vi "setConfiguration.vi"(8 "error in (no error)":errorcluster, 10 "configuration":T2={"exposure_time_s"=nan, "delay_time_s"=nan, "roi"={"x0"=18446744073709551615, "y0"=18446744073709551615, "x1"=18446744073709551615, "y1"=18446744073709551615}, "timestamp_mode"=65535, "pixelrate"=4294967295, "conversion_factor"=0.7, "trigger_mode"=65535, "acquire_mode"=65535, "acquire_sequence_number"=1, "metadata_mode"=65535, "noisefilter_mode"=65535, "pixel_format"=0, "binning"={"vert"=0, "horz"=0, "mode"=0}, "auto_exposure"={"region"=0, "min_exposure_s"=0.001, "max_exposure_s"=0.1}} {"conversion_factor" format="%.2g"; "auto_exposure"."region" items=["balanced", "center_based", "corner_based", "full", "custom"]; "binning"."mode" items=["sum", "average"]; "noisefilter_mode" items=["Undefined"=65535, "OFF"=0, "ON"=1]; "exposure_time_s" format="%#_6f"; "timestamp_mode" items=["Undefined"=65535, "OFF"=0, "Binary"=1, "Binary+ASCII"=2, "ASCII"=3]; "acquire_mode" items=["Undefined"=65535, "auto"=0, "external"=1, "external modulate"=2]; "trigger_mode" items=["Undefined"=65535, "auto sequence"=0, "software trigger"=1, "external exposure start & software trigger"=2, "external exposure control"=3, "external synchronized"=4, "fast external exposure control"=5, "external CDS control"=6, "slow external exposure control"=7, "external synchronized HDSDI"=258]; "metadata_mode" items=["Undefined"=65535, "OFF"=0, "ON"=1]}, 11 "Camera in":refnum<class "Camera.lvclass">) -> (0 "error out":errorcluster, 3 "Camera out":refnum<class "Camera.lvclass">)   [LabVIEW 2019, in "Camera.lvclass"]
doc: "Sets a new coniguration to the camera."
uses:
  Camera.lvclass
  Camera.lvclass/Camera.ctl
  pco.sdk/TimingControl/TimingControl.lvlib
  pco.sdk/ImageSensor/ImageSensor.lvlib
  pco.sdk/RecordingControl/RecordingControl.lvlib
  pco.sdk/CameraDescription/CameraDescription.lvlib
  pco.sdk/GeneralCameraControl/GeneralCameraControl.lvlib
  Controls/binning.ctl
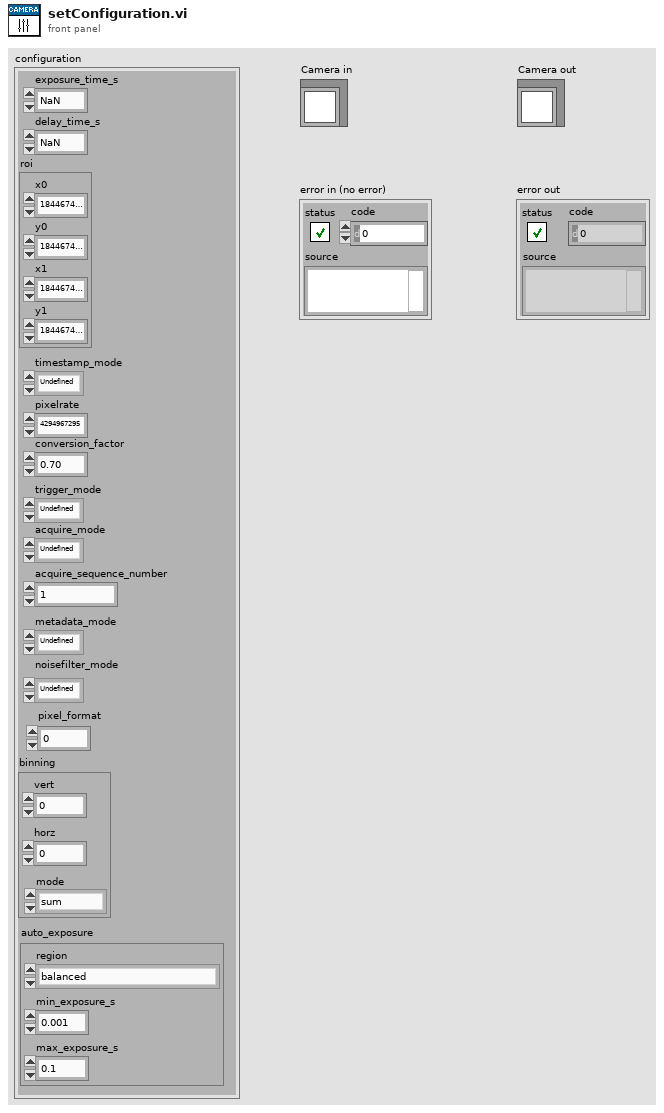
[diagram p1: front panel]
types:
  T1 = typedef "Camera.lvclass/binning.ctl" = cluster{"vert":u16, "horz":u16, "mode":u16}
  T2 = cluster{"exposure_time_s":dbl, "delay_time_s":dbl, "roi":cluster{"x0":u64, "y0":u64, "x1":u64, "y1":u64}, "timestamp_mode":u16, "pixelrate":u32, "conversion_factor":sgl, "trigger_mode":u16, "acquire_mode":u16, "acquire_sequence_number":u32, "metadata_mode":u16, "noisefilter_mode":u16, "pixel_format":u32, "binning":T1, "auto_exposure":cluster{"region":u16, "min_exposure_s":dbl, "max_exposure_s":dbl}}
  T3 = cluster{"region":u16, "min_exposure_s":dbl, "max_exposure_s":dbl}
  T4 = cluster{"wSensorTypeDESC":u16, "wSensorSubTypeDESC":u16, "wMaxHorzResStdDESC":u16, "wMaxVertResStdDESC":u16, "wMaxHorzResExtDESC":u16, "wMaxVertResExtDESC":u16, "wDynResDESC":u16, "wMaxBinHorzDESC":u16, "wBinHorzSteppingDESC":u16, "wMaxBinVertDESC":u16, "wBinVertSteppingDESC":u16, "wRoiHorStepsDESC":u16, "wRoiVertStepsDESC":u16, "wNumADCsDESC":u16, "wMinSizeHorzDESC":u16, "dwPixelRateDESC":u32[], "wConvFactDESC":u16[], "sCoolingSetpoints":i16[], "wSoftRoiHorStepsDESC":u16, "wSoftRoiVertStepsDESC":u16, "wIRDESC":u16, "wMinSizeVertDESC":u16, "dwMinDelayDESC":u32, "dwMaxDelayDESC":u32, "dwMinDelayStepDESC":u32, "dwMinExposureDESC":u32, "dwMaxExposureDESC":u32, "dwMinExposureStepDESC":u32, "dwMinDelayIRDESC":u32, "dwMaxDelayIRDESC":u32, "dwMinExposureIRDESC":u32, "dwMaxExposureIRDESC":u32, "wTimeTableDESC":u16, "wDoubleImageDESC":u16, "sMinCoolSetDESC":i16, "sMaxCoolSetDESC":i16, "sDefaultCoolSetDESC":i16, "wPowerDownModeDESC":u16, "wOffsetRegulationDESC":u16, "wColorPatternDESC":u16, "wPatternTypeDESC":u16, "wNumCoolingSetpoints":u16, "dwGeneralCapsDESC1":u32, "dwGeneralCapsDESC2":u32, "dwExtSyncFrequency":u32[], "dwGeneralCapsDESC3":u32, "dwGeneralCapsDESC4":u32}
  T5 = enum16{"SETUP_TYPE_SHUTTERMODE", "SETUP_TYPE_PIXELFORMAT", "SETUP_TYPE_SENSOR_DYNRES"}
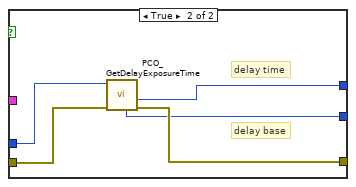
[diagram p4: hidden frame]
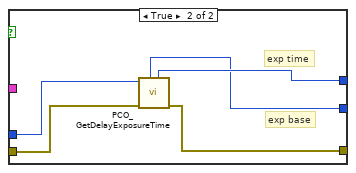
[diagram p5: hidden frame]
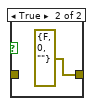
[diagram p9: hidden frame]
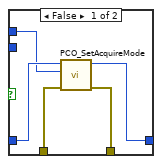
[diagram p12: hidden frame]
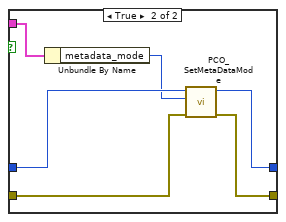
[diagram p13: hidden frame]
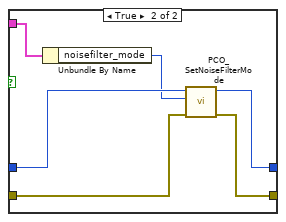
[diagram p14: hidden frame]
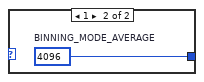
[diagram p16: hidden frame]
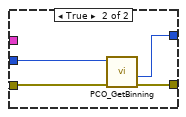
[diagram p17: hidden frame]
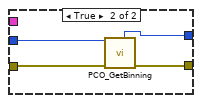
[diagram p18: hidden frame]
diagram:
  n1 = case shown="No Error" "error in (no error)" {
    selector: "error in (no error)" -> [w10 w448]
    tunnel: [w13 w448] -> w4
    tunnel: [w12 w447] -> w2
    tunnel: "Camera in" -> [w11 w447]
    tunnel: "configuration" -> [w6 _]
    frame No Error {
      n2 = call-dynamic "isRecording.vi"("Camera in"=w11, "error in (no error)"=w10) -> ("Camera out"=w7:refnum<class "Camera.lvclass">, "recording"=w9:bool, "error out"=w8:errorcluster)  [unwired: 11 in]
      n3 = case shown="False" w9 {
        tunnel: [w18 errorcluster {"status"=TRUE, "code"=-2146029534, "source"="Cannot set configuration\nif recording is running!"} ("error constant")] -> w13
        tunnel: [w17 w445] -> w12
        tunnel: w8 -> [w16 _]
        tunnel: w7 -> [w14 w445]
        tunnel: w6 -> [w15 _]
        frame False {
          n4 = Unbundle By Name(w14) -> ("camera_handle"=w19:u64)
          n5 = Not Equal To 0?(x=w19) -> (x != 0?=w20:bool)
          n6 = case shown="True" w20 {
            tunnel: [errorcluster {"status"=TRUE, "code"=1, "source"="In set_configuration:\nCamera handle is zero"} ("error constant") w36] -> w18
            tunnel: w19 -> [_ w63]
            tunnel: w16 -> [_ w62]
            tunnel: w14 -> [w21 w27]
            tunnel: [w21 w28] -> w17
            tunnel: w15 -> [_ w61]
            frame False {
            }
            frame True {
              n7 = flat-sequence {
                tunnel: w63 -> [w70]
                tunnel: w62 -> [w67]
                tunnel: w61 -> [w66]
                tunnel: [w66] -> w60
                tunnel: [w65] -> w59
                tunnel: [w64] -> w58
                tunnel: w60 -> [w117]
                tunnel: w59 -> [w116]
                tunnel: w58 -> [w115]
                tunnel: [w117] -> w57
                tunnel: [w114] -> w56
                tunnel: [w113] -> w55
                tunnel: w57 -> [w145]
                tunnel: w56 -> [w144]
                tunnel: w55 -> [w143]
                tunnel: w27 -> [w150]
                tunnel: [w145] -> w54
                tunnel: [w142] -> w53
                tunnel: [w141] -> w52
                tunnel: w54 -> [w165]
                tunnel: w53 -> [w164]
                tunnel: w52 -> [w163]
                tunnel: [w165] -> w51
                tunnel: [w162] -> w49
                tunnel: [w161] -> w47
                tunnel: w51 -> [w188]
                tunnel: [w188] -> w50
                tunnel: w49 -> [w187]
                tunnel: [w185] -> w48
                tunnel: w47 -> [w186]
                tunnel: [w184] -> w46
                tunnel: w50 -> [w205]
                tunnel: w48 -> [w208]
                tunnel: w46 -> [w207]
                tunnel: w27 -> [w206]
                tunnel: [w205] -> w45
                tunnel: [w204] -> w44
                tunnel: [w203] -> w43
                tunnel: w27 -> [w200]
                tunnel: w45 -> [w242]
                tunnel: w27 -> [w247]
                tunnel: w44 -> [w246]
                tunnel: w43 -> [w245]
                tunnel: [w242] -> w42
                tunnel: [w241] -> w41
                tunnel: [w240] -> w40
                tunnel: w42 -> [w271]
                tunnel: w41 -> [w273]
                tunnel: w40 -> [w272]
                tunnel: [w271] -> w39
                tunnel: [w270] -> w38
                tunnel: [w269] -> w37
                tunnel: w27 -> [w262]
                tunnel: w39 -> [w284]
                tunnel: w38 -> [w300]
                tunnel: w37 -> [w299]
                tunnel: [w284] -> w35
                tunnel: [w296] -> w34
                tunnel: [w295] -> w33
                tunnel: w27 -> [w293]
                tunnel: w35 -> [w345]
                tunnel: w34 -> [w347]
                tunnel: w33 -> [w342]
                tunnel: w27 -> [w346]
                tunnel: [w340] -> w23
                tunnel: [w345] -> w32
                tunnel: [w347] -> w31
                tunnel: [w341] -> w30
                tunnel: w32 -> [w353]
                tunnel: w31 -> [w361]
                tunnel: w30 -> [w360]
                tunnel: [w353] -> w26
                tunnel: [w352] -> w25
                tunnel: [w348] -> w24
                tunnel: [w431] -> w29
                tunnel: [w434] -> _
                tunnel: w26 -> [w434]
                tunnel: w25 -> [w432]
                tunnel: w24 -> [w433]
                tunnel: w23 -> [w430]
                frame #0 {
                  w73 = nan
                  # "Set Delay and Exposure Time"
                  n8 = Unbundle By Name(w66) -> ("exposure_time_s"=w74:dbl, "delay_time_s"=w72:dbl)
                  n9 = Not Equal?(x=w73, y=w74) -> (x != y?=w68:bool)
                  n10 = Not Equal?(x=w73, y=w72) -> (x != y?=w69:bool)
                  n11 = Or(x=w68, y=w69) -> (x .or. y?=w71:bool)
                  n12 = case shown="True" w71 {
                    tunnel: w66 -> [_ w88]
                    tunnel: w70 -> [w76 w86]
                    tunnel: w69 -> [_ w89]
                    tunnel: w68 -> [_ w91]
                    tunnel: w67 -> [w75 w87]
                    tunnel: [w76 w78] -> w65
                    tunnel: [w75 w77] -> w64
                    frame False {
                    }
                    frame True {
                      # "If delay time is nan"
                      # "If exp time is nan"
                      n13 = Not(x=w89) -> (.not. x?=w90:bool)
                      n14 = Not(x=w91) -> (.not. x?=w92:bool)
                      n15 = case shown="False" w90 {
                        tunnel: w86 -> [_ w101]
                        tunnel: w88 -> [w96 _]
                        tunnel: [w95 w99] -> w80
                        tunnel: [w94 w98] -> w79
                        tunnel: w87 -> [w93 w102]
                        tunnel: [w93 w100] -> w83
                        frame False {
                          # "delay base"
                          # "delay time"
                          n16 = Unbundle By Name(w96) -> ("delay_time_s"=w97:dbl)
                          n17 = call "calcTimeBase.vi"("time"=w97) -> ("base_calculated"=w94:u16, "time_calculated"=w95:u32)  [unwired: 9 in]
                        }
                        frame True {
                          # "delay base"
                          # "delay time"
                          n18 = call "PCO_GetDelayExposureTime.vi"("error in (no error)"=w102, "ph"=w101) -> ("error out"=w100:errorcluster, "dwDelay"=w99:u32, "wTimeBaseDelay"=w98:u16)  [unwired: 3 in, 4 out]
                        }
                      }
                      n19 = case shown="False" w92 {
                        tunnel: w86 -> [_ w112]
                        tunnel: w88 -> [w107 _]
                        tunnel: [w105 w109] -> w82
                        tunnel: [w104 w108] -> w81
                        tunnel: w87 -> [w103 w111]
                        tunnel: [w103 w110] -> w84
                        frame False {
                          # "exp base"
                          # "exp time"
                          n20 = Unbundle By Name(w107) -> ("exposure_time_s"=w106:dbl)
                          n21 = call "calcTimeBase.vi"("time"=w106) -> ("base_calculated"=w104:u16, "time_calculated"=w105:u32)  [unwired: 9 in]
                        }
                        frame True {
                          # "exp base"
                          # "exp time"
                          n22 = call "PCO_GetDelayExposureTime.vi"("error in (no error)"=w111, "ph"=w112) -> ("error out"=w110:errorcluster, "dwExposure"=w109:u32, "wTimeBaseExposure"=w108:u16)  [unwired: 3 in, 4 out]
                        }
                      }
                      n23 = Merge Errors(w84, w83) -> (w85:errorcluster)
                      n24 = call "PCO_SetDelayExposureTime.vi"("wTimeBaseExposure"=w81, "wTimeBaseDelay"=w79, "error in (no error)"=w85, "dwExposure"=w82, "dwDelay"=w80, "ph"=w86) -> ("error out"=w77:errorcluster, "ph out"=w78:u64)  [unwired: 3 in, 1 out]
                    }
                  }
                }
                frame #1 {
                  w127 = u64 18446744073709551615
                  # "Set ROI"
                  n25 = Unbundle By Name(w117) -> ("roi.x0"=w126:u64, "roi.y0"=w125:u64, "roi.x1"=w124:u64, "roi.y1"=w123:u64)
                  n26 = Not Equal?(x=w127, y=w126) -> (x != y?=w122:bool)
                  n27 = Not Equal?(x=w127, y=w125) -> (x != y?=w121:bool)
                  n28 = Not Equal?(x=w127, y=w124) -> (x != y?=w120:bool)
                  n29 = Not Equal?(x=w127, y=w123) -> (x != y?=w119:bool)
                  n30 = Compound Arithmetic op=AND(w122, w121, w120, w119) -> (w118:bool)
                  n31 = case shown="True" w118 {
                    tunnel: w117 -> [_ w136]
                    tunnel: w116 -> [w129 w134]
                    tunnel: w115 -> [w128 w135]
                    tunnel: [w129 w138] -> w114
                    tunnel: [w128 w137] -> w113
                    frame False {
                    }
                    frame True {
                      n32 = Unbundle By Name(w136) -> ("roi.x0"=w133:u64, "roi.y0"=w132:u64, "roi.x1"=w131:u64, "roi.y1"=w130:u64)
                      n33 = call "PCO_SetROI.vi"("ph"=w134, "wRoiX0"=w133, "wRoiX1"=w131, "error in (no error)"=w135, "wRoiY0"=w132, "wRoiY1"=w130) -> ("ph out"=w138:u64, "error out"=w137:errorcluster)  [unwired: 7 in, 1 out]
                    }
                  }
                }
                frame #2 {
                  w139 = u32 256 ("camera_description.dwGeneralCapsDESC1")
                  # "Set Timestamp Mode"
                  # "GENERALCAPS1_NO_TIMESTAMP"
                  n34 = Unbundle By Name(w150) -> ("dwGeneralCapsDESC1"=w149:u32)
                  n35 = Unbundle By Name(w145) -> ("timestamp_mode"=w151:u16)
                  n36 = Not Equal?(x=u16 65535 ("timestamp_mode"), y=w151) -> (x != y?=w148:bool)
                  n37 = And(x=w149, y=w139) -> (x .and. y?=w140:u32)
                  n38 = Not Equal?(x=w140, y=w139) -> (x != y?=w147:bool)
                  n39 = And(x=w148, y=w147) -> (x .and. y?=w146:bool)
                  n40 = case shown="True" w146 {
                    tunnel: w145 -> [_ w160]
                    tunnel: w144 -> [w154 w159]
                    tunnel: w143 -> [w153 w158]
                    tunnel: [w154 w156] -> w142
                    tunnel: [w153 w155] -> w141
                    frame False {
                    }
                    frame True {
                      n41 = Unbundle By Name(w160) -> ("timestamp_mode"=w157:u16)
                      n42 = call "PCO_SetTimestampMode.vi"("error in (no error)"=w158, "wTimeStampMode"=w157, "ph"=w159) -> ("error out"=w155:errorcluster, "ph out"=w156:u64)  [unwired: 6 in, 1 out]
                    }
                  }
                }
                frame #3 {
                  # "Set Pixelrate"
                  n43 = Unbundle By Name(w165) -> ("pixelrate"=w168:u32)
                  n44 = Not Equal?(x=u32 4294967295 ("pixelrate"), y=w168) -> (x != y?=w166:bool)
                  n45 = case shown="True" w166 {
                    tunnel: w165 -> [_ w181]
                    tunnel: w164 -> [w170 w180]
                    tunnel: w163 -> [w169 w178]
                    tunnel: [w170 w172] -> w162
                    tunnel: [w169 w171] -> w161
                    frame False {
                    }
                    frame True {
                      w175 = -2147479520 ("ErrorMessage")
                      # "Ignore\nPCO_ERROR_FIRMWARE_NOT_SUPPORTED"
                      n46 = Unbundle By Name(w181) -> ("pixelrate"=w179:u32)
                      n47 = call "PCO_SetPixelRate.vi"("error in (no error)"=w178, "dwPixelRate"=w179, "ph"=w180) -> ("error out"=w173:errorcluster, "ErrorMessage"=w177:i32, "ph out"=w172:u64)  [unwired: 6 in]
                      n48 = And(x=w177, y=w175) -> (x .and. y?=w176:i32)
                      n49 = Equal?(x=w176, y=w175) -> (x = y?=w174:bool)
                      n50 = case shown="False" w174 {
                        tunnel: w173 -> [w182 _]
                        tunnel: [w182 errorcluster {"status"=FALSE, "code"=0, "source"=""} ("error out")] -> w171
                        frame False {
                        }
                        frame True {
                        }
                      }
                    }
                  }
                }
                frame #4 {
                  # "Set Trigger Mode"
                  n51 = Unbundle By Name(w188) -> ("trigger_mode"=w190:u16)
                  n52 = Not Equal?(x=u16 65535 ("timestamp_mode"), y=w190) -> (x != y?=w189:bool)
                  n53 = case shown="True" w189 {
                    tunnel: w188 -> [_ w199]
                    tunnel: w187 -> [w193 w198]
                    tunnel: w186 -> [w192 w197]
                    tunnel: [w193 w195] -> w185
                    tunnel: [w192 w194] -> w184
                    frame False {
                    }
                    frame True {
                      n54 = Unbundle By Name(w199) -> ("trigger_mode"=w196:u16)
                      n55 = call "PCO_SetTriggerMode.vi"("error in (no error)"=w197, "wTriggerMode"=w196, "ph"=w198) -> ("error out"=w194:errorcluster, "ph out"=w195:u64)  [unwired: 6 in, 1 out]
                    }
                  }
                }
                frame #5 {
                  w201 = u32 512 ("camera_description.dwGeneralCapsDESC1")
                  # "Set Acquire Mode"
                  # "GENERALCAPS1_NO_ACQUIREMODE"
                  n56 = Unbundle By Name(w206) -> ("dwGeneralCapsDESC1"=w212:u32)
                  n57 = Unbundle By Name(w205) -> ("acquire_mode"=w213:u16)
                  n58 = Not Equal?(x=u16 65535 ("timestamp_mode"), y=w213) -> (x != y?=w211:bool)
                  n59 = And(x=w212, y=w201) -> (x .and. y?=w202:u32)
                  n60 = Not Equal?(x=w202, y=w201) -> (x != y?=w210:bool)
                  n61 = And(x=w211, y=w210) -> (x .and. y?=w209:bool)
                  n62 = case shown="True" w209 {
                    tunnel: w205 -> [_ w228]
                    tunnel: w208 -> [w216 w227]
                    tunnel: w207 -> [w215 w226]
                    tunnel: [w216 w224] -> w204
                    tunnel: [w215 w223] -> w203
                    tunnel: w200 -> [_ w222]
                    frame False {
                    }
                    frame True {
                      w219 = u32 2097152 ("y")
                      # "GENERALCAPS1_EXT_ACQUIRE"
                      n63 = Unbundle By Name(w222) -> ("dwGeneralCapsDESC1"=w221:u32)
                      n64 = Unbundle By Name(w228) -> ("acquire_mode"=w225:u16, "acquire_sequence_number"=w218:u32)
                      n65 = And(x=w221, y=w219) -> (x .and. y?=w220:u32)
                      n66 = Equal?(x=w220, y=w219) -> (x = y?=w217:bool)
                      n67 = case shown="True" w217 {
                        tunnel: w227 -> [w233 w235]
                        tunnel: w226 -> [w232 w238]
                        tunnel: w225 -> [w231 w239]
                        tunnel: [w230 w236] -> w224
                        tunnel: [w229 w237] -> w223
                        tunnel: w218 -> [_ w234]
                        frame False {
                          n68 = call "PCO_SetAcquireMode.vi"("error in (no error)"=w232, "wAcquMode"=w231, "ph"=w233) -> ("error out"=w229:errorcluster, "ph out"=w230:u64)  [unwired: 6 in, 1 out]
                        }
                        frame True {
                          n69 = call "PCO_SetAcquireModeEx.vi"("error in (no error)"=w238, "dwNumberImages"=w234, "wAcquMode"=w239, "ph"=w235) -> ("error out"=w237:errorcluster, "ph out"=w236:u64)  [unwired: 5 in, 1 out]
                        }
                      }
                    }
                  }
                }
                frame #6 {
                  w243 = u32 16384 ("camera_description.dwGeneralCapsDESC1")
                  # "Set Metadata Mode"
                  # "GENERALCAPS1_METADATA"
                  n70 = Unbundle By Name(w247) -> ("dwGeneralCapsDESC1"=w251:u32)
                  n71 = Unbundle By Name(w242) -> ("metadata_mode"=w252:u16)
                  n72 = Not Equal?(x=u16 65535 ("timestamp_mode"), y=w252) -> (x != y?=w250:bool)
                  n73 = And(x=w251, y=w243) -> (x .and. y?=w244:u32)
                  n74 = Equal?(x=w244, y=w243) -> (x = y?=w249:bool)
                  n75 = And(x=w250, y=w249) -> (x .and. y?=w248:bool)
                  n76 = case shown="False" w248 {
                    tunnel: w242 -> [_ w261]
                    tunnel: w246 -> [w255 w260]
                    tunnel: w245 -> [w254 w259]
                    tunnel: [w255 w257] -> w241
                    tunnel: [w254 w256] -> w240
                    frame False {
                    }
                    frame True {
                      n77 = Unbundle By Name(w261) -> ("metadata_mode"=w258:u16)
                      n78 = call "PCO_SetMetaDataMode.vi"("error in (no error)"=w259, "wMetaDataMode"=w258, "ph"=w260) -> ("error out"=w256:errorcluster, "ph out"=w257:u64)  [unwired: 4 in, 3 out]
                    }
                  }
                }
                frame #7 {
                  w266 = u32 1 ("camera_description.dwGeneralCapsDESC1")
                  # "GENERALCAPS1_NOISE_FILTER"
                  # "Set Noise Filter Mode"
                  n79 = Unbundle By Name(w262) -> ("dwGeneralCapsDESC1"=w268:u32)
                  n80 = Unbundle By Name(w271) -> ("noisefilter_mode"=w274:u16)
                  n81 = Not Equal?(x=u16 65535 ("timestamp_mode"), y=w274) -> (x != y?=w265:bool)
                  n82 = And(x=w268, y=w266) -> (x .and. y?=w267:u32)
                  n83 = Equal?(x=w267, y=w266) -> (x = y?=w264:bool)
                  n84 = And(x=w265, y=w264) -> (x .and. y?=w263:bool)
                  n85 = case shown="False" w263 {
                    tunnel: w271 -> [_ w283]
                    tunnel: w273 -> [w277 w282]
                    tunnel: w272 -> [w276 w281]
                    tunnel: [w277 w279] -> w270
                    tunnel: [w276 w278] -> w269
                    frame False {
                    }
                    frame True {
                      n86 = Unbundle By Name(w283) -> ("noisefilter_mode"=w280:u16)
                      n87 = call "PCO_SetNoiseFilterMode.vi"("error in (no error)"=w281, "wNoiseFilterMode"=w280, "ph"=w282) -> ("error out"=w278:errorcluster, "ph out"=w279:u64)  [unwired: 6 in, 1 out]
                    }
                  }
                }
                frame #8 {
                  w290 = u16 1 ("x")
                  w301 = u16 65535 ("timestamp_mode")
                  # "Check if binning is changable"
                  # "Set Binning"
                  n88 = Unbundle By Name(w293) -> ("wMaxBinHorzDESC"=w292:u16, "wMaxBinVertDESC"=w291:u16)
                  n89 = Unbundle By Name(w284) -> ("binning.vert"=w303:u16, "binning.horz"=w302:u16, "binning.mode"=w294:u16)
                  n90 = Not Equal?(x=w301, y=w303) -> (x != y?=w298:bool)
                  n91 = Not Equal?(x=w301, y=w302) -> (x != y?=w297:bool)
                  n92 = Not Equal?(x=w290, y=w292) -> (x != y?=w288:bool)
                  n93 = Not Equal?(x=w290, y=w291) -> (x != y?=w289:bool)
                  n94 = Or(x=w298, y=w297) -> (x .or. y?=w286:bool)
                  n95 = Or(x=w288, y=w289) -> (x .or. y?=w287:bool)
                  n96 = And(x=w287, y=w286) -> (x .and. y?=w285:bool)
                  n97 = case shown="True" w285 {
                    tunnel: w300 -> [w305 w312]
                    tunnel: w299 -> [w304 w319]
                    tunnel: [w305 w313] -> w296
                    tunnel: [w304 w314] -> w295
                    tunnel: w298 -> [_ w323]
                    tunnel: w297 -> [_ w322]
                    tunnel: w284 -> [_ w318]
                    tunnel: w294 -> [_ w311]
                    frame False {
                    }
                    frame True {
                      # "If bin horz is nan"
                      # "If bin vert is nan"
                      n98 = Not(x=w323) -> (.not. x?=w321:bool)
                      n99 = Not(x=w322) -> (.not. x?=w320:bool)
                      n100 = case shown="False" w321 {
                        tunnel: w318 -> [w335 _]
                        tunnel: [w333 w336] -> w310
                        tunnel: w319 -> [w334 w339]
                        tunnel: [w334 w338] -> w316
                        tunnel: w312 -> [_ w337]
                        frame False {
                          n101 = Unbundle By Name(w335) -> ("binning.vert"=w333:u16)
                        }
                        frame True {
                          n102 = call "PCO_GetBinning.vi"("error in (no error)"=w339, "ph"=w337) -> ("error out"=w338:errorcluster, "wBinVert"=w336:u16)  [unwired: 5 in, 3 out]
                        }
                      }
                      n103 = case shown="0, Default" w311 {
                        tunnel: [w324 w325] -> w308
                        frame 0, Default {
                          w324 = u16 0  # BINNING_MODE_SUM
                        }
                        frame 1 {
                          w325 = u16 4096  # BINNING_MODE_AVERAGE
                        }
                      }
                      n104 = case shown="False" w320 {
                        tunnel: w318 -> [w328 _]
                        tunnel: [w326 w329] -> w309
                        tunnel: w312 -> [_ w332]
                        tunnel: w319 -> [w327 w331]
                        tunnel: [w327 w330] -> w317
                        frame False {
                          n105 = Unbundle By Name(w328) -> ("binning.horz"=w326:u16)
                        }
                        frame True {
                          n106 = call "PCO_GetBinning.vi"("error in (no error)"=w331, "ph"=w332) -> ("error out"=w330:errorcluster, "wBinHorz"=w329:u16)  [unwired: 5 in, 3 out]
                        }
                      }
                      n107 = Or(x=w308, y=w309) -> (x .or. y?=w307:u16)
                      n108 = Or(x=w310, y=w308) -> (x .or. y?=w306:u16)
                      n109 = Merge Errors(w316, w317) -> (w315:errorcluster)
                      n110 = call "PCO_SetBinning.vi"("error in (no error)"=w315, "wBinVert"=w306, "wBinHorz"=w307, "ph"=w312) -> ("error out"=w314:errorcluster, "ph out"=w313:u64)  [unwired: 5 in, 1 out]
                    }
                  }
                }
                frame #9 {
                  n111 = Unbundle By Name(w345) -> ("auto_exposure"=w344:T3)
                  n112 = Bundle By Name(cluster=w346, "auto_exposure"=w344) -> (w343:refnum<class "Camera.lvclass">)
                  n113 = call "updateAutoExposure.vi"("error in (no error)"=w342, "Camera in"=w343) -> ("error out"=w341:errorcluster, "Camera out"=w340:refnum<class "Camera.lvclass">)  [unwired: 8 in]
                }
                frame #10 {
                  # "Camera can be switched to different pixelformat output"
                  # "uint GENERALCAPS3_CAMERA_SETUP_PIXELFORMAT = 0x00020000"
                  n114 = call "PCO_GetCameraDescription.vi"("error in (no error)"=w360, "ph"=w361) -> ("error out"=w355:errorcluster, "strDescription"=w359:T4, "ph out"=w356:u64)  [unwired: 6 in, 1 out]
                  n115 = Unbundle By Name(w353) -> ("pixel_format"=w350:u32)
                  n116 = Unbundle By Name(w359) -> ("wDynResDESC"=w354:u16, "dwGeneralCapsDESC3"=w358:u32)
                  n117 = Not Equal?(x=w350, y=u32 4294967295) -> (x != y?=w349:bool)
                  n118 = And(x=w358, y=u32 131072) -> (x .and. y?=w363:u32)
                  n119 = Not Equal To 0?(x=w363) -> (x != 0?=w357:bool)
                  n120 = case shown="True" w349 {
                    tunnel: w357 -> [_ w372]
                    tunnel: w356 -> [w364 w371]
                    tunnel: w355 -> [w365 w370]
                    tunnel: w354 -> [_ w369]
                    tunnel: [w365 w368] -> w352
                    tunnel: w350 -> [_ w367]
                    tunnel: [w364 w366] -> w348
                    frame False {
                    }
                    frame True {
                      n121 = case shown="False" w372 {
                        tunnel: w370 -> [w379 w395]
                        tunnel: [w378 w391] -> w368
                        tunnel: w371 -> [w373 w394]
                        tunnel: w369 -> [w380 _]
                        tunnel: w367 -> [w376 w388]
                        tunnel: [w373 w385] -> w366
                        frame False {
                          n122 = call "dynResToPixelFormat.vi"("error in (no error)"=w379, "dyn_res"=w380) -> ("error out"=w374:errorcluster, "PixelFormat"=w377:u32)  [unwired: 8 in]
                          n123 = Equal?(x=w376, y=w377) -> (x = y?=w375:bool)
                          n124 = case shown="False" w375 {
                            tunnel: [w381 w384] -> w378
                            tunnel: w374 -> [w383 w384]
                            frame False {
                              n125 = Merge Errors(errorcluster {"status"=TRUE, "code"=-1609170943, "source"="Unsupported pixel format"} ("error constant"), w383) -> (w381:errorcluster)
                            }
                            frame True {
                            }
                          }
                        }
                        frame True {
                          w386 = T5."SETUP_TYPE_PIXELFORMAT" ("wTypeIn")
                          n126 = call "PCO_GetCameraSetup.vi"("error in (no error)"=w395, "wTypeIn"=w386, "ph"=w394) -> ("error out"=w393:errorcluster, "ph out"=w392:u64, "dwSetup"=w387:u32[])  [unwired: 4 in, 2 out]
                          n127 = Index Array(array=w387, index=1) -> (element=w389:u32)
                          n128 = case shown="No Error" w393 {
                            selector: w393 -> [w401 w421]
                            tunnel: w392 -> [w403 w419]
                            tunnel: [w400 w420] -> w391
                            tunnel: w389 -> [w405 _]
                            tunnel: w388 -> [w398 _]
                            tunnel: w387 -> [w399 _]
                            tunnel: w386 -> [w397 _]
                            tunnel: [w396 w419] -> w385
                            frame No Error {
                              n129 = And(x=w398, y=w405) -> (x .and. y?=w404:u32)
                              n130 = Not Equal To 0?(x=w404) -> (x != 0?=w402:bool)
                              n131 = case shown="False" w402 {
                                tunnel: w403 -> [w406 w415]
                                tunnel: w401 -> [w408 w412]
                                tunnel: [w407 w411] -> w400
                                tunnel: w399 -> [_ w418]
                                tunnel: w398 -> [_ w416]
                                tunnel: w397 -> [_ w413]
                                tunnel: [w406 w410] -> w396
                                frame False {
                                n132 = Merge Errors(errorcluster {"status"=TRUE, "code"=-1609170943, "source"="Unsupported pixel format"} ("error constant"), w408) -> (w407:errorcluster)
                                }
                                frame True {
                                n133 = Replace Array Subset(array=w418, new element=w416, index=0) -> (w414:u32[])
                                n134 = call "PCO_SetCameraSetup.vi"("error in (no error)"=w412, "dwSetup"=w414, "wType"=w413, "ph"=w415) -> ("error out"=w411:errorcluster, "ph out"=w410:u64)  [unwired: 5 in, 1 out]
                                }
                              }
                            }
                            frame Error {
                              n135 = Bundle By Name(cluster=w421, "status"=TRUE, "source"="Unsupported pixel format") -> (w420:errorcluster)
                            }
                          }
                        }
                      }
                    }
                  }
                }
                frame #11 {
                  # "Determine if the requested conversion factor is one of the allowed values from the camera description"
                  n136 = Unbundle By Name(w430) -> ("wConvFactDESC"=w426:u16[])
                  n137 = Unbundle By Name(w434) -> ("conversion_factor"=w427:sgl)
                  n138 = Multiply(x=w427, y=sgl 100.0) -> (x*y=w425:sgl)
                  n139 = Equal?(x=w426, y=w425) -> (x = y?=w429:bool[])
                  n140 = Or Array Elements(Boolean array=w429) -> (logical OR=w428:bool)
                  n141 = case shown="True" w428 {
                    tunnel: w433 -> [_ w444]
                    tunnel: w432 -> [w436 w443]
                    tunnel: [w435 w442] -> w431
                    tunnel: w427 -> [_ w441]
                    frame False {
                      n142 = Merge Errors(errorcluster {"status"=TRUE, "code"=-1609170943, "source"="Conversion factor not supported"} ("error constant"), w436) -> (w435:errorcluster)
                    }
                    frame True {
                      n143 = Multiply(x=w441, y=sgl 100.0) -> (x*y=w439:sgl)
                      n144 = To Unsigned Word Integer(number=w439) -> (unsigned 16bit integer=w438:u16)
                      n145 = call "PCO_SetConversionFactor.vi"("error in (no error)"=w443, "wConvFact"=w438, "ph"=w444) -> ("error out"=w442:errorcluster)  [unwired: 6 in, 2 out]
                    }
                  }
                }
              }
              n146 = call-dynamic "armCamera.vi"("Camera in"=w23, "error in (no error)"=w29) -> ("Camera out"=w28:refnum<class "Camera.lvclass">, "error out"=w36:errorcluster)  [unwired: 12 in]
            }
          }
        }
        frame True {
        }
      }
    }
    frame Error {
    }
  }
  "error out" <- w4
  "Camera out" <- w2
